vi "Render Picture.vi"(11 "Line In":refnum<class "Line example.lvclass">) -> (1 "Picture":picture, 3 "Line Out":refnum<class "Line example.lvclass">)   [LabVIEW 2023, in "Line example.lvclass"]
doc: "Render the line into the picture."
uses:
  Line example.lvclass
  Line example.lvclass/Line example.ctl
  Point/Point.lvclass
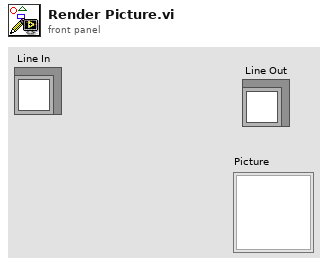
[diagram p1: front panel]
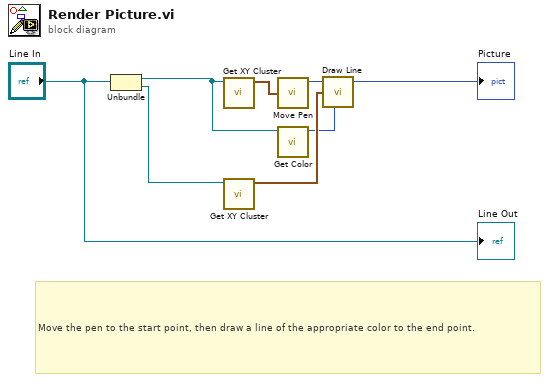
[diagram p0: block diagram]
diagram:
  # "Move the pen to the start point, then draw a line of the appropriate color to the end point."
  n1 = Unbundle("Line In") -> (w3:refnum<class "Point.lvclass">, w6:refnum<class "Point.lvclass">)
  n2 = call "Get XY Cluster.vi"("Point.lvclass"=w3) -> ("XY Cluster"=w7:cluster{"X":i16, "Y":i16})  [unwired: 10 in]
  n3 = call "Get XY Cluster.vi"("Point.lvclass"=w6) -> ("XY Cluster"=w4:cluster{"X":i16, "Y":i16})  [unwired: 10 in]
  n4 = call <vilib>:"Move Pen.vi"("new position"=w7) -> ("new picture"=w5:picture)  [unwired: 2 in, 2 out]
  n5 = call "Get Color.vi"("Point"=w3) -> ("Color"=w2:u32)  [unwired: 10 in]
  n6 = call <vilib>:"Draw Line.vi"("picture"=w5, "end point"=w4, "color(black)"=w2) -> ("new picture"=→"Picture":picture)  [unwired: 2 in, 4 out]
  "Line Out" <- "Line In"
